vi "SetPieceArray.vi"(8 "error in (no error)":errorcluster, 10 "pieceArray":refnum<class "Piece.lvclass">[][](array[class]), 11 "object in":refnum<class "Board.lvclass">) -> (0 "error out":errorcluster, 3 "object out":refnum<class "Board.lvclass">)   [LabVIEW 2020]
uses:
  Board.lvclass
  Pieces/Piece.lvclass
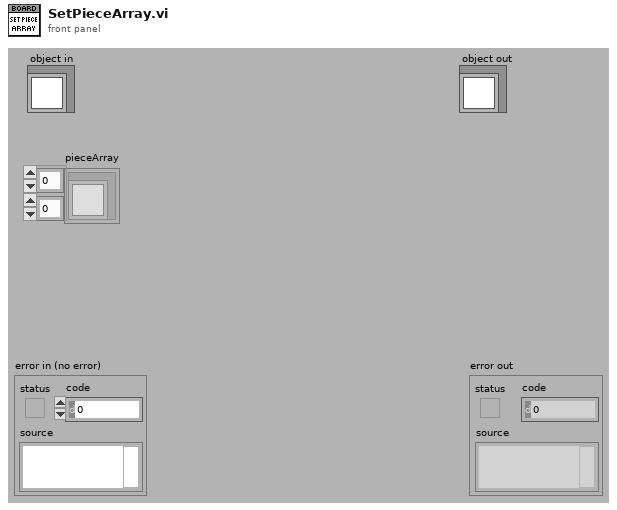
[diagram p1: front panel]
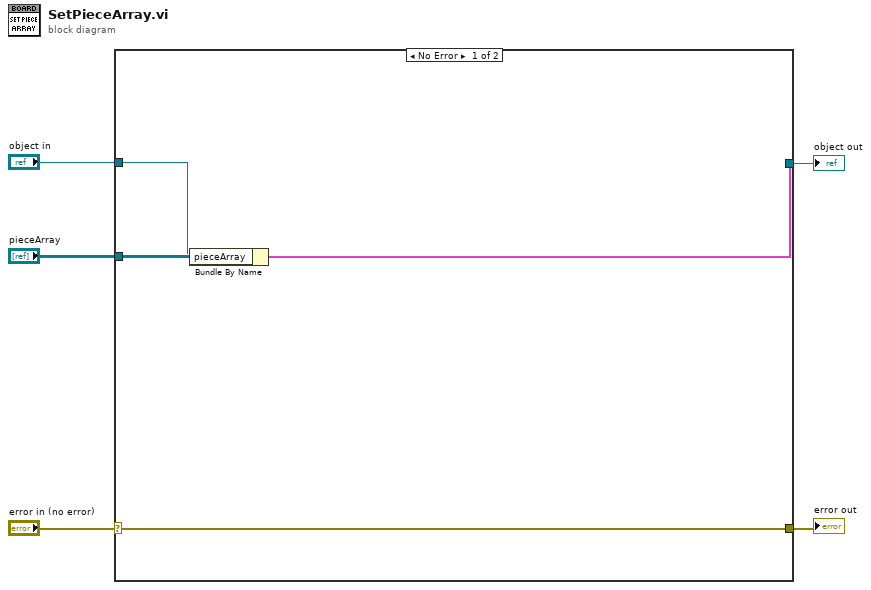
[diagram p0: block diagram]
diagram:
  n1 = case shown="No Error" "error in (no error)" {
    selector: "error in (no error)" -> [w8 w11]
    tunnel: [w8 w11] -> w4
    tunnel: [w6 w10] -> w2
    tunnel: "object in" -> [w7 w10]
    tunnel: "pieceArray" -> [w9 _]
    frame No Error {
      n2 = Bundle By Name(cluster=w7, "pieceArray"=w9) -> (w6:cluster{})
    }
    frame Error {
    }
  }
  "error out" <- w4
  "object out" <- w2
